vi "Change Recipe Label.vi"(8 "error in (no error)":errorcluster, 10 "New Label":string, 11 "Recipe Window in":refnum<class "Recipe Window.lvclass">) -> (0 "error out":errorcluster, 3 "Recipe Window out":refnum<class "Recipe Window.lvclass">)   [LabVIEW 2021, in "Recipe.lvlib" / "Recipe Window.lvclass"]
uses:
  Recipe Window.lvclass
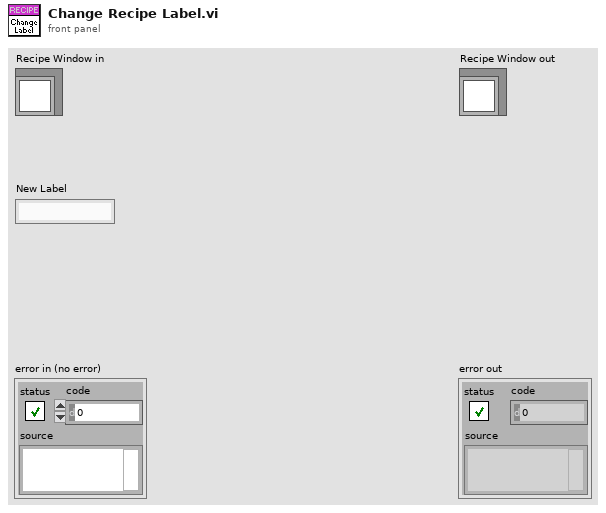
[diagram p1: front panel]
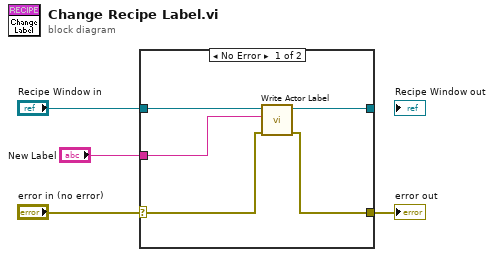
[diagram p0: block diagram]
diagram:
  n1 = case shown="No Error" "error in (no error)" {
    selector: "error in (no error)" -> [w6 w11]
    tunnel: [w5 w11] -> w3
    tunnel: [w9 w10] -> _
    tunnel: "Recipe Window in" -> [w8 w10]
    tunnel: "New Label" -> [w7 _]
    frame No Error {
      n2 = call-dynamic "Write Actor Label.vi"("error in (no error)"=w6, "Actor Label"=w7, "Monitored Actor in"=w8) -> ("error out"=w5:errorcluster, "Monitored Actor out"=w9:refnum<class "Recipe Window.lvclass">)  [unwired: 7 in]
    }
    frame Error {
    }
  }
  "error out" <- w3
